vi "Factory Create.vi"(8 "Error In":errorcluster, 11 "reference in":refnum<class "Configuration Base.lvclass">) -> (0 "Error Out":errorcluster, 3 "reference out":refnum<class "Configuration Base.lvclass">)   [LabVIEW 2023, in "HAL GOOP4.lvlib" / "Configuration Base.lvclass"]
uses:
  Configuration Base.lvclass
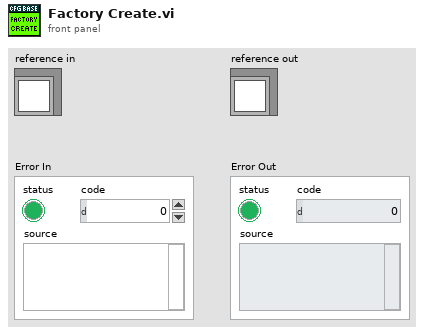
[diagram p1: front panel]
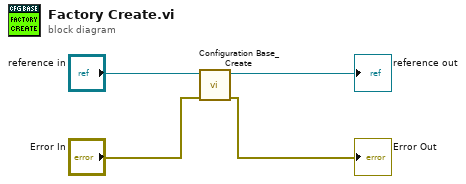
[diagram p0: block diagram]
diagram:
  n1 = call "Configuration Base_Create.vi"("Error In"="Error In", "reference in"="reference in") -> ("Error Out"=→"Error Out":errorcluster, "reference out"=→"reference out":refnum<class "Configuration Base.lvclass">)  [unwired: 8 in]
